vi "Untitled 10.vi"() -> ()   [LabVIEW 2019]
panel:
  out "date/time string 3":string
  out "time stamp":timestamp
  out "double precision float":dbl
  out "date/time string 2":string
  out "date/time string":string
  out "Time":string
  out "UTC Time":string
  out "date/time":string
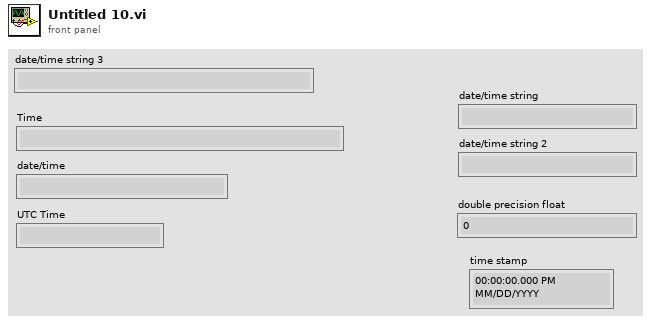
[diagram p1: front panel]
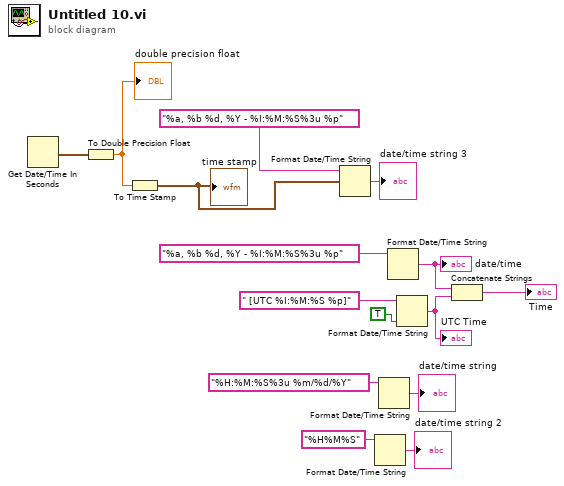
[diagram p0: block diagram]
diagram:
  n1 = Get Date/Time In Seconds() -> (seconds since 1Jan1904=w6:timestamp)
  n2 = To Double Precision Float(number=w6) -> (double precision float=w5:dbl)
  "double precision float" <- w5
  n3 = To Time Stamp(1:w5) -> (0:w3:timestamp)
  "time stamp" <- w3
  n4 = Format Date/Time String(time format string (%c)="%a, %b %d, %Y - %I:%M:%S%3u %p", seconds (now)=w3) -> (date/time string=→"date/time string 3":string)  [unwired: 1 in]
  n5 = Format Date/Time String(time format string (%c)="%H%M%S") -> (date/time string=→"date/time string 2":string)  [unwired: 2 in]
  n6 = Format Date/Time String(time format string (%c)="%H:%M:%S%3u %m/%d/%Y") -> (date/time string=→"date/time string":string)  [unwired: 2 in]
  n7 = Format Date/Time String(time format string (%c)="%a, %b %d, %Y - %I:%M:%S%3u %p") -> (date/time string=w11:string)  [unwired: 2 in]
  "date/time" <- w11
  n8 = Format Date/Time String(time format string (%c)=" [UTC %I:%M:%S %p]", UTC format=TRUE) -> (date/time string=w12:string)  [unwired: 1 in]
  "UTC Time" <- w12
  n9 = Concatenate Strings(w11, w12) -> (→"Time":string)
